vi "PathToINIBroadcast.vi"(8 "error in (no error)":errorcluster, 10 "PathToINI":path, 11 "ModuleID":i32) -> (0 "error out":errorcluster)   [LabVIEW 2014, in "SpecAnPlugins.lvlib" / "SpecAnBase.lvclass"]
uses:
  SpecAnBase.lvclass
  SpecAnModule/PublicAPI/Requests/clEventType.ctl
  <vilib>/Utility/error.llb/Error Cluster From Error Code.vi
  <vilib>/ErrorRing/Error Ring.xnode
  SpecAnModule/SpecAnModule.lvlib
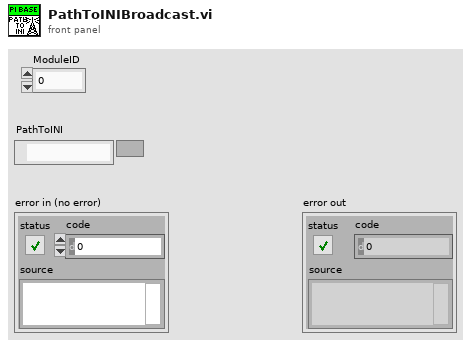
[diagram p1: front panel]
types:
  T1 = typedef "SpecAnModule.lvlib/clBroadcastEvents.ctl" = cluster{"DidInit":refnum<user-event>, "StatusUpdate":refnum<user-event>, "ErrorReport":refnum<user-event>, "DidStop":refnum<user-event>, "PathToINI":refnum<user-event>, "TraceName":refnum<user-event>}
  T2 = typedef "SpecAnModule.lvlib/clEventType.ctl" = cluster{"ModuleID":i32, "Data":variant}
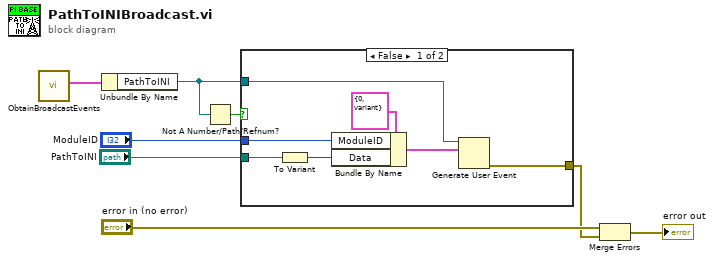
[diagram p0: block diagram]
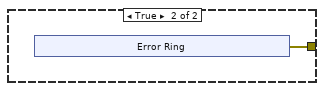
[diagram p2: hidden frame]
diagram:
  n1 = call "ObtainBroadcastEvents.vi"() -> ("clBroadcastEvents"=w8:T1)  [unwired: 10 in, 1 out]
  n2 = Unbundle By Name(w8) -> ("PathToINI"=w2:refnum<user-event>)
  n3 = Not A Number/Path/Refnum?(number/path/refnum=w2) -> (NaN/Path/Refnum?=w3:bool)
  n4 = case shown="False" w3 {
    tunnel: "ModuleID" -> [w14 _]
    tunnel: "PathToINI" -> [w12 _]
    tunnel: w2 -> [w10 _]
    tunnel: [w9 w16] -> w1
    frame False {
      n5 = To Variant(anything=w12) -> (Variant=w13:variant)
      n6 = Bundle By Name(cluster=T2 {"ModuleID"=0, "Data"=variant} ("clEventType"), "ModuleID"=w14, "Data"=w13) -> (w11:T2)
      n7 = Generate User Event(user event=w10, event data cluster=w11) -> (error out=w9:errorcluster)  [unwired: 2 in, 1 out]
    }
    frame True {
      n8 = xnode "Error Ring"() -> ("error out"=w16:errorcluster)
    }
  }
  n9 = Merge Errors("error in (no error)", w1) -> (→"error out":errorcluster)
